vi "Save_File_Dialog.vi"(8 "error in (no error)":errorcluster, 11 "Filename":string) -> (0 "error out":errorcluster, 2 "Cancelled":bool, 3 "Path":path)   [LabVIEW 2013]
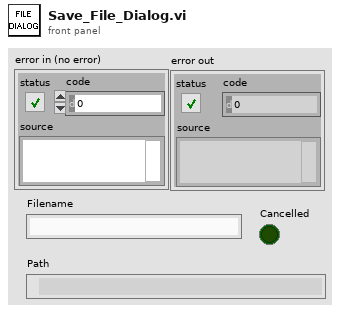
[diagram p1: front panel]
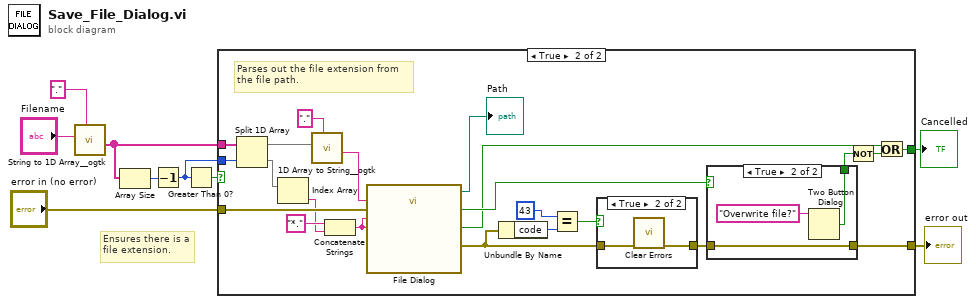
[diagram p0: block diagram]
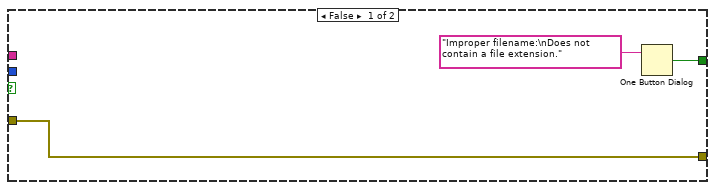
[diagram p2: hidden frame]
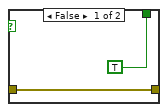
[diagram p4: hidden frame]
diagram:
  # "Ensures there is a\nfile extension."
  n1 = call <userlib>:"String to 1D Array__ogtk.vi"("delimiter (Tab)"=".", "string"="Filename") -> ("Array of Strings"=w3:string[])  [unwired: 9 in]
  n2 = Array Size(array=w3) -> (size(s)=w2:i32)
  n3 = Decrement(x=w2) -> (x-1=w1:i32)
  n4 = Greater Than 0?(x=w1) -> (x > 0?=w4:bool)
  n5 = case shown="True" w4 {
    tunnel: "error in (no error)" -> [w12 w27]
    tunnel: [w11 w26] -> w8
    tunnel: [w12 w24] -> w7
    tunnel: w3 -> [_ w23]
    tunnel: w1 -> [_ w22]
    frame False {
      n6 = One Button Dialog(message="Improper filename:\nDoes not contain a file extension.") -> (true=w11:bool)  [unwired: 1 in]
    }
    frame True {
      # "Parses out the file extension from\nthe file path."
      n7 = Split 1D Array(array=w23, index=w22) -> (first subarray=w21:string[], second subarray=w18:string[])
      n8 = Index Array(array=w18) -> (element=w15:string)  [unwired: 1 in]
      n9 = call <userlib>:"1D Array to String__ogtk.vi"("delimiter (Tab)"=".", "Array of Strings"=w21) -> ("delimited string"=w19:string)  [unwired: 9 in]
      n10 = Concatenate Strings("*." ("string"), w15) -> (w16:string)
      n11 = call "File Dialog"("default name"=w19, "error in"=w27, "pattern (all files)"=w16, "pattern label"=w16) -> ("selected path"=→"Path":path, "exists"=w28:bool, "cancelled"=w14:bool, "error out"=w33:errorcluster)  [unwired: 8 in]
      n12 = Unbundle By Name(w33) -> ("code"=w30:i32)
      n13 = Equal?(x=43, y=w30) -> (x = y?=w32:bool)
      n14 = case shown="True" w32 {
        tunnel: w33 -> [w35 w37]
        tunnel: [w35 w36] -> w34
        frame False {
        }
        frame True {
          n15 = call <vilib>:"Clear Errors.vi"("error in (no error)"=w37) -> ("error out"=w36:errorcluster)  [unwired: 6 in]
        }
      }
      n16 = case shown="True" w28 {
        tunnel: [w39 w42] -> w24
        tunnel: w34 -> [w39 w42]
        tunnel: [TRUE ("T button?") w41] -> w29
        frame False {
        }
        frame True {
          n17 = Two Button Dialog(message="Overwrite file?") -> (T button?=w41:bool)  [unwired: 2 in]
        }
      }
      n18 = Not(x=w29) -> (.not. x?=w13:bool)
      n19 = Or(x=w14, y=w13) -> (x .or. y?=w26:bool)
    }
  }
  "error out" <- w7
  "Cancelled" <- w8
